vi "Abort Acquisition.vi"(8 "error in (no error)":errorcluster, 11 "CCDCamera in":refnum<class "iKon-L.lvclass">) -> (0 "error out":errorcluster, 3 "CCDCamera out":refnum<class "iKon-L.lvclass">)   [LabVIEW 2018, in "iKon-L.lvclass"]
doc: "Abort the current acquisition\n\nThis function should be used carefully."
uses:
  iKon-L.lvclass
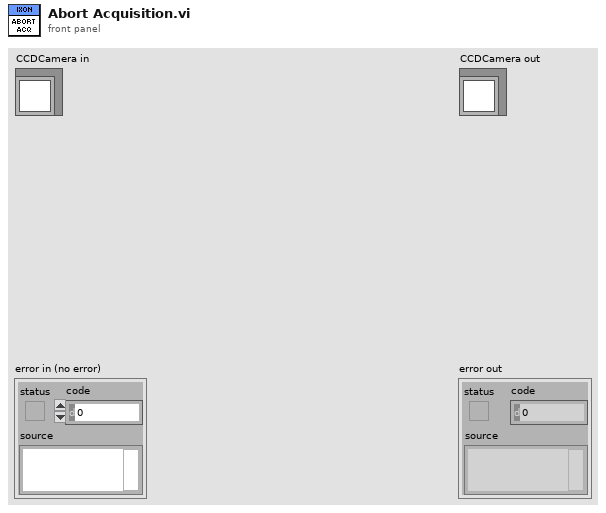
[diagram p1: front panel]
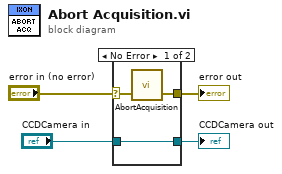
[diagram p0: block diagram]
diagram:
  n1 = case shown="No Error" "error in (no error)" {
    selector: "error in (no error)" -> [w5 w8]
    tunnel: [w7 w8] -> w3
    tunnel: "CCDCamera in" -> [w6 w9]
    tunnel: [w6 w9] -> w2
    frame No Error {
      n2 = call <userlib>:"AbortAcquisition.vi"("error in (no error)"=w5) -> ("error out"=w7:errorcluster)  [unwired: 1 in, 1 out]
    }
    frame Error {
    }
  }
  "error out" <- w3
  "CCDCamera out" <- w2
